vi "SEH Init.vi"(8 "error in (no error)":errorcluster, 10 "Number of Priorities":i32=3, 11 "Notifications per Priority":i32=5) -> (0 "error out":errorcluster)   [LabVIEW 2014]
doc: "This VI initializes the notification queue used to transfer errors from Specific Error Handler instances to the Central Error Handler. \n\nThe notification queue is a priority queue where each priority has a fixed number of entries. Elements are always removed from the highest priority available. Priorities are specified in a lowest-to-highest order, so priority 0 is the highest priority and priority Number of Priorities-1 is the lowest.\n\nYou only need to call this VI if you are using error notification."
uses:
  Controls/Shared/SEH Error Notification Command.ctl
  Controls/Shared/SEH Error Notification Config.ctl
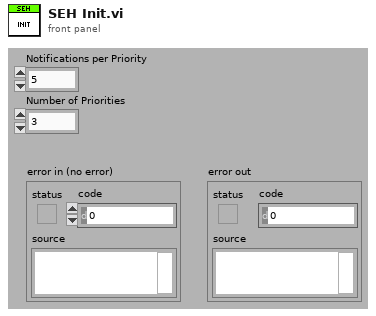
[diagram p1: front panel]
types:
  T1 = typedef "SEH Error Notification Config.ctl" = cluster{"Number of Priorities":i32, "Notifications per Priority":i32}
  T2 = typedef "SEH Error Notification Command.ctl" = enum16{"Init", "Send Error", "Check Error", "Invalid Command"}
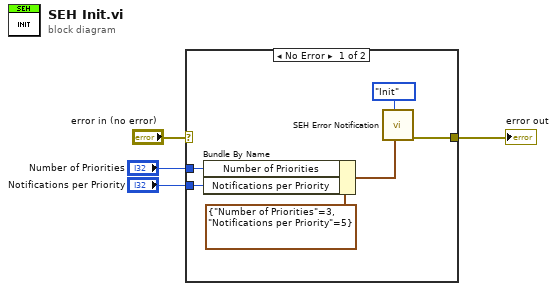
[diagram p0: block diagram]
diagram:
  n1 = case shown="No Error" "error in (no error)" {
    selector: "error in (no error)" -> [_ w11]
    tunnel: "Number of Priorities" -> [w7 _]
    tunnel: "Notifications per Priority" -> [w6 _]
    tunnel: [w5 w11] -> w1
    frame No Error {
      n2 = Bundle By Name(cluster=T1 {"Number of Priorities"=3, "Notifications per Priority"=5} ("Configuration"), "Number of Priorities"=w7, "Notifications per Priority"=w6) -> (w8:T1)
      n3 = call "SEH Error Notification.vi"("Configuration"=w8, "Command"=SEH_Error_Notification_Command."Init") -> ("Transmission Error"=w5:errorcluster)  [unwired: 4 in, 5 out]
    }
    frame Error {
    }
  }
  "error out" <- w1
